vi "SDG Check for Global Channel Ports.vi"(0 "Global Channel In":refnum<k21>, 11 "error in (no error)":errorcluster) -> (4 "Global Channel Out":refnum<k21>, 15 "error out":errorcluster)   [LabVIEW 2021, in "DAQ_Static Digital State Generation.lvlib"]
doc: "Checks for the presence of port in the global channel input and throws the required error when identified."
uses:
  DAQ_Static Digital State Generation.lvlib
  <vilib>/Utility/error.llb/Error Cluster From Error Code.vi
  <vilib>/ErrorRing/Error Ring.xnode
  <resource>/objmgr/daqmx.rc
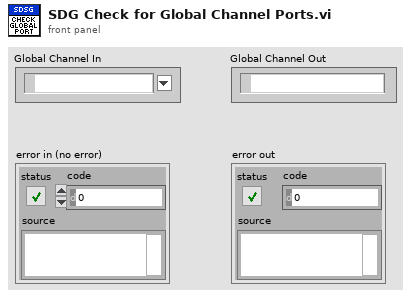
[diagram p1: front panel]
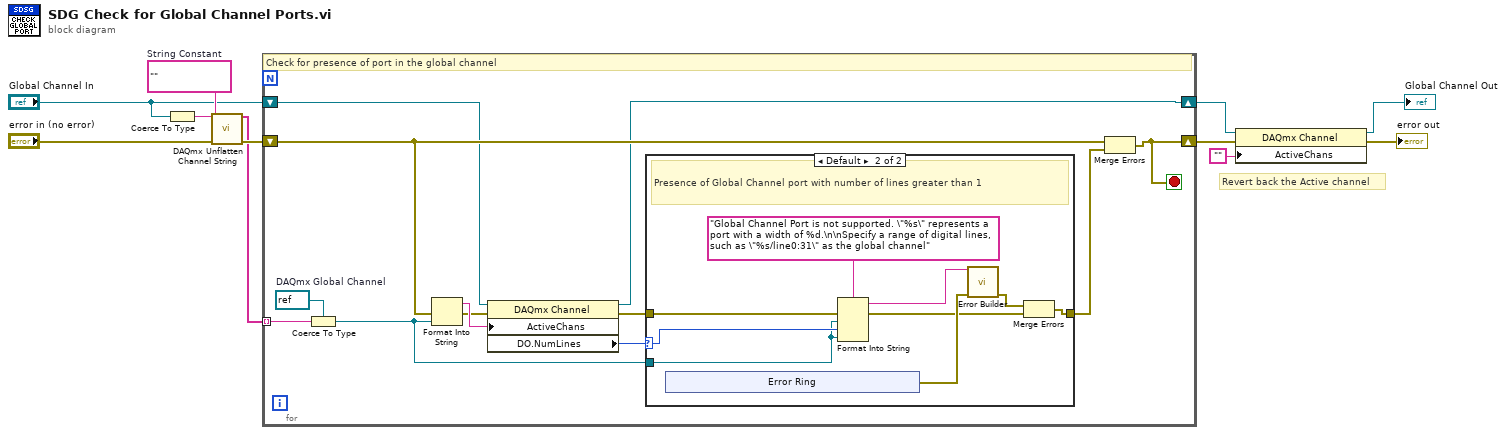
[diagram p0: block diagram]
diagram:
  w3 = ""  # String Constant
  # "Revert back the Active channel"
  n1 = Coerce To Type(0:"Global Channel In", 1:w3) -> (2:w1:string)
  n2 = call <vilib>:"DAQmx Unflatten Channel String.vi"("names in"=w1, "error in"="error in (no error)") -> ("names out"=w9:string[], "error out"=w10:errorcluster)  [unwired: 12 in]
  n3 = for {
    tunnel: w9 -> [w23] mode=indexing
    shift-right: [w20] -> w6
    shift-left: w10 -> [w16]
    shift-right: [w12] -> w8
    shift-left: "Global Channel In" -> [w13]
    stop <- w20 stop-if-true
    w22 = refnum<k21> refnum  # DAQmx Global Channel
    # "Check for presence of port in the global channel"
    n4 = Coerce To Type(0:w23, 1:w22) -> (2:w17:refnum<k21>)
    n5 = Format Into String(error in=w16, w17) -> (resulting string=w15:string, error out=w14:errorcluster)  [unwired: 2 in]
    n6 = property class="DAQmx Channel"(reference=w13, error in=w14, "ActiveChans"=w15) -> (reference out=w12:refnum<k21>, error out=w18:errorcluster, "DO.NumLines"=w19:u32)
    n7 = case shown="Default" w19 {
      selector: w19 -> [_ w27]
      tunnel: [w24 w25] -> w21
      tunnel: w17 -> [_ w26]
      tunnel: w18 -> [w24 w28]
      frame 1 {
        # "The current active channel is a singe digital line"
      }
      frame Default {
        # "Presence of Global Channel port with number of lines greater than 1"
        n8 = xnode "Error Ring"() -> ("error out"=w32:errorcluster)
        n9 = Format Into String(format string="Global Channel Port is not supported. \"%s\" represents a port with a width of %d.\n\nSpecify a range of digital lines, such as \"%s/line0:31\" as the global channel" ("error message (\"\")"), error in=w28, w26, w27, w26) -> (resulting string=w33:string, error out=w30:errorcluster)  [unwired: 1 in]
        n10 = call "Error Builder.vi"("Error String"=w33, "Error In"=w32) -> ("Error Out"=w31:errorcluster)  [unwired: 13 in]
        n11 = Merge Errors(w31, w30) -> (w25:errorcluster)
      }
    }
    n12 = Merge Errors(w16, w21) -> (w20:errorcluster)
  }
  n13 = property class="DAQmx Channel"(reference=w8, error in=w6, "ActiveChans"="") -> (reference out=→"Global Channel Out":refnum<k21>, error out=→"error out":errorcluster)
